vi "Read One DAQ Waveform.vi"(7 "Offset in":u32, 8 "error in (no error)":errorcluster, 9 "Total Length":u32, 10 "Waveform Datatype in":T1, 11 "CIF_CIPC_Fifo_U8 in":refnum<class "CIF_CIPC_Fifo_DAQ.lvclass">) -> (0 "error out":errorcluster, 1 "Done":bool, 2 "Waveform Datatype out":T1, 3 "CIF_CIPC_Fifo_U8 out":refnum<class "CIF_CIPC_Fifo_DAQ.lvclass">, 4 "Timeout":bool, 5 "Offset out":u32)   [LabVIEW 2021, in "CIF_CIPC_Fifo_DAQ.lvclass"]
uses:
  ChannelCommon/typedef/Datatype Waveform.ctl
  <vilib>/CIF Foundation/CIF CIPC/SubVIs/Check Error.vi
  <vilib>/CIF Foundation/CIF CIPC/SubVIs/Notify Of New Write.vi
  <vilib>/CIF Foundation/CIF CIPC/SubVIs/Get dll Path.vi
  <vilib>/CIF Foundation/CIF CIPC/SubVIs/Get Element Write Position.vi
  <vilib>/Utility/error.llb/Trim Whitespace.vi
  <vilib>/Utility/error.llb/Error Cluster From Error Code.vi
  CIF_CIPC_Fifo_DAQ.lvclass
  CIF_CIPC_Fifo_DAQ.lvclass/CIF_CIPC_Fifo_DAQ.ctl
  <vilib>/CIF Foundation/CIF CIPC/TypeDefs/Read Position.ctl
  <vilib>/CIF Foundation/CIF CIPC/CIF_NI_CIPC.lvlib
  <vilib>/CIF Foundation/CIF CIPC/TypeDefs/Read Configuration.ctl
  <vilib>/CIF Foundation/CIF CIPC/TypeDefs/Data Element Details.ctl
  ChannelCommon/typedef/Waveform Metadata.ctl
  ChannelCommon/ChannelCommon.lvlib
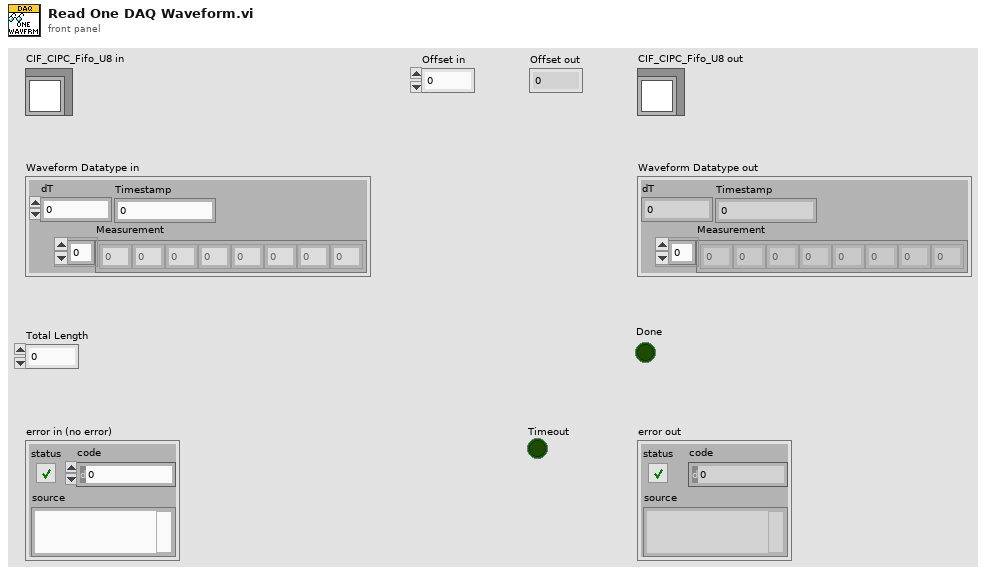
[diagram p1: front panel]
types:
  T1 = typedef "ChannelCommon.lvlib/Datatype Waveform.ctl" = cluster{"Measurement":dbl[], "dT":dbl, "Timestamp":i64}
  T2 = typedef "ChannelCommon.lvlib/Waveform Metadata.ctl" = cluster{"Timestamp":i64, "dT":dbl, "Array Length":u64}
  T3 = typedef "CIF_NI_CIPC.lvlib/Data Element Details.ctl" = cluster{"Bytes to Read":u32, "Element Offset":u32}
  T4 = typedef "CIF_NI_CIPC.lvlib/Read Configuration.ctl" = cluster{"Read Position":T5, "Element Offset":i32, "Prepend Array Size":bool, "Get Read Position":bool}
  T5 = typedef "CIF_NI_CIPC.lvlib/Read Position.ctl" = enum16{"Next", "Newest", "Oldest", "Next Available", "Absolute"}
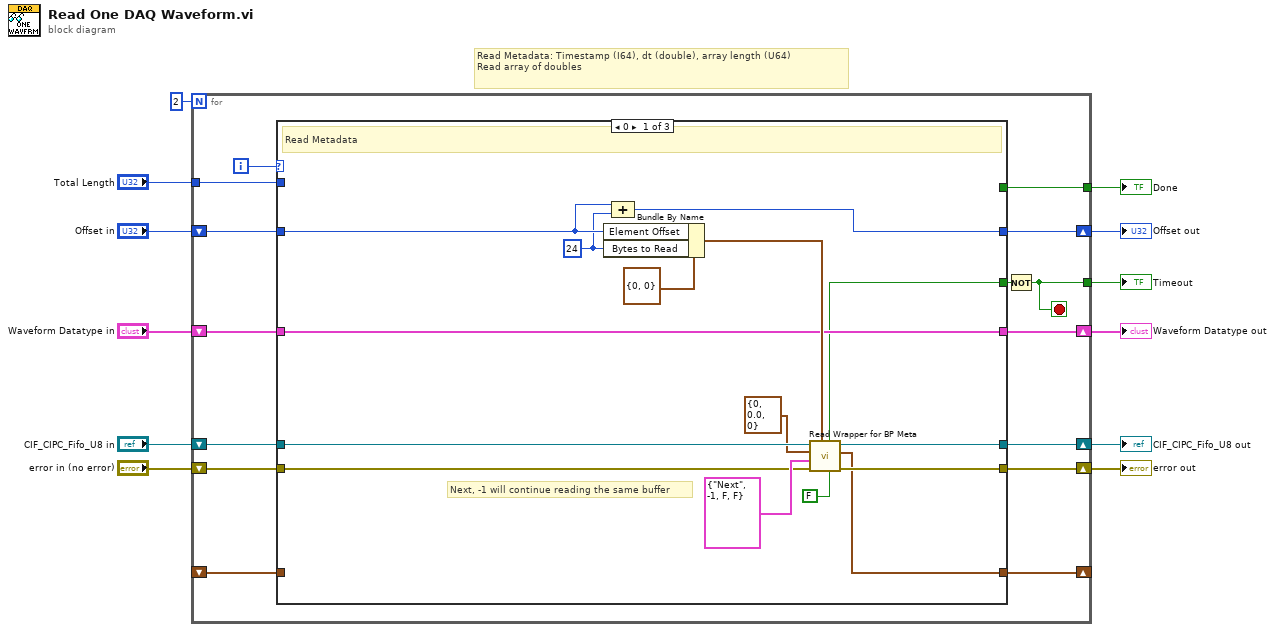
[diagram p0: block diagram]
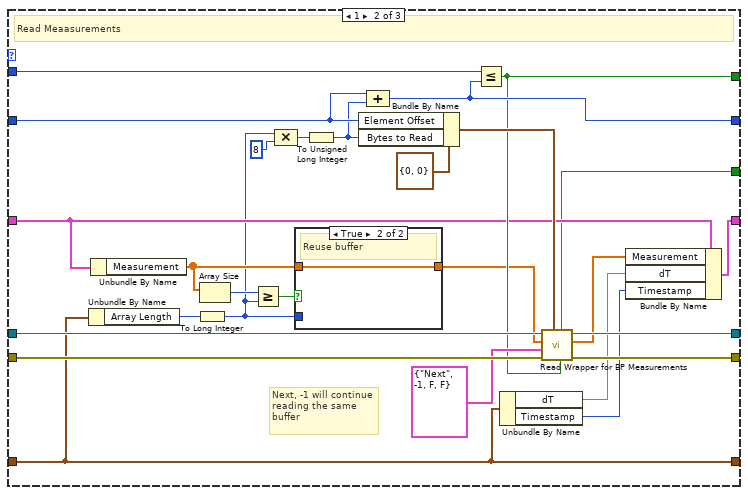
[diagram p2: hidden frame]
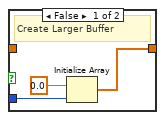
[diagram p3: hidden frame]
diagram:
  # "Read Metadata: Timestamp (I64), dt (double), array length (U64)\nRead array of doubles"
  n1 = for {
    N: 2 -> [_]
    shift-right: [w26] -> w11
    shift-left: "CIF_CIPC_Fifo_U8 in" -> [w27]
    shift-right: [w18] -> w5
    shift-left: "Waveform Datatype in" -> [w23]
    shift-right: [w21] -> w3
    shift-left: "error in (no error)" -> [w22]
    shift-right: [w20] -> w4
    shift-left: "Offset in" -> [w25]
    shift-right: [w19] -> _
    shift-left: _ -> [w15]
    tunnel: "Total Length" -> [w17]
    tunnel: [w16] -> w6
    tunnel: [w13] -> w1
    i -> [w24]
    stop <- w13 stop-if-true
    n2 = case shown="0" w24 {
      tunnel: w27 -> [w41 w62 w76]
      tunnel: [w40 w65 w76] -> w26
      tunnel: w25 -> [w33 w68 w78]
      tunnel: w23 -> [w29 w51 w77]
      tunnel: w22 -> [w37 w67 w75]
      tunnel: [w36 w64 w75] -> w21
      tunnel: [w31 w60 w78] -> w20
      tunnel: [w30 w54 w74] -> w19
      tunnel: [w29 w55 w77] -> w18
      tunnel: w17 -> [_ w61 _]
      tunnel: [_ w59 _] -> w16
      tunnel: w15 -> [_ w54 w74]
      tunnel: [w28 w43 _] -> w14
      frame 0 {
        w32 = u32 24 ("Bytes to Read")
        # "Next, -1 will continue reading the same buffer"
        # "Read Metadata"
        n3 = Bundle By Name(cluster=T3 {"Bytes to Read"=0, "Element Offset"=0} ("Data Element"), "Element Offset"=w33, "Bytes to Read"=w32) -> (w35:T3)
        n4 = Compound Arithmetic op=ADD(w33, w32) -> (w31:u32)
        n5 = call "Read Wrapper for BP Meta.vi"("Last Read"=FALSE, "Data Element"=w35, "error in (no error)"=w37, "Read Configuration"=T4 {"Read Position"=enum."Next", "Element Offset"=-1, "Prepend Array Size"=FALSE, "Get Read Position"=FALSE}, "Waveform Metadata in"=T2 {"Timestamp"=0, "dT"=0.0, "Array Length"=0} ("Waveform Meta Data"), "CIF_CIPC_Fifo_U8 in"=w41) -> ("error out"=w36:errorcluster, "Waveform Metadata out"=w30:T2, "CIF_CIPC_Fifo_U8 out"=w40:refnum<class "CIF_CIPC_Fifo_DAQ.lvclass">, "Success"=w28:bool)  [unwired: 1 in, 1 out]
      }
      frame 1 {
        # "Next, -1 will continue reading the same buffer"
        # "Read Meaasurements"
        n6 = Unbundle By Name(w54) -> ("Array Length"=w49:u64)
        n7 = Unbundle By Name(w51) -> ("Measurement"=w50:dbl[])
        n8 = To Long Integer(number=w49) -> (32bit integer=w48:i32)
        n9 = Array Size(array=w50) -> (size(s)=w52:i32)
        n10 = Greater Or Equal?(x=w52, y=w48) -> (x >= y?=w53:bool)
        n11 = Compound Arithmetic op=MULTIPLY(w48, 8 ("value")) -> (w47:i32)
        n12 = case shown="True" w53 {
          tunnel: w50 -> [_ w73]
          tunnel: [w72 w73] -> w44
          tunnel: w48 -> [w70 _]
          frame False {
            # "Create Larger Buffer"
            n13 = Initialize Array(0.0, w70) -> (w72:dbl[])
          }
          frame True {
            # "Reuse buffer"
          }
        }
        n14 = To Unsigned Long Integer(number=w47) -> (unsigned 32bit integer=w45:u32)
        n15 = Bundle By Name(cluster=T3 {"Bytes to Read"=0, "Element Offset"=0} ("Data Element"), "Element Offset"=w68, "Bytes to Read"=w45) -> (w66:T3)
        n16 = Compound Arithmetic op=ADD(w68, w45) -> (w60:u32)
        n17 = Less Or Equal?(x=w61, y=w60) -> (x <= y?=w59:bool)
        n18 = Unbundle By Name(w54) -> ("dT"=w57:dbl, "Timestamp"=w56:i64)
        n19 = call "Read Wrapper for BP Measurements.vi"("Last Read"=w59, "Data Element"=w66, "error in (no error)"=w67, "Read Configuration"=T4 {"Read Position"=enum."Next", "Element Offset"=-1, "Prepend Array Size"=FALSE, "Get Read Position"=FALSE}, "Data in"=w44, "CIF_CIPC_Fifo_U8 in"=w62) -> ("error out"=w64:errorcluster, "Data out"=w58:dbl[], "CIF_CIPC_Fifo_U8 out"=w65:refnum<class "CIF_CIPC_Fifo_DAQ.lvclass">, "Success"=w43:bool)  [unwired: 1 in, 1 out]
        n20 = Bundle By Name(cluster=w51, "Measurement"=w58, "dT"=w57, "Timestamp"=w56) -> (w55:T1)
      }
      frame 2, Default {
        # "Default case"
      }
    }
    n21 = Not(x=w14) -> (.not. x?=w13:bool)
  }
  "Offset out" <- w4
  "error out" <- w3
  "Waveform Datatype out" <- w5
  "CIF_CIPC_Fifo_U8 out" <- w11
  "Done" <- w6
  "Timeout" <- w1
